vi "Append Text polymorphic.vi"   [LabVIEW 2019]
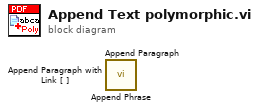
[diagram p0: block diagram]
diagram:
  n1 = call <userlib>:"Append Phrase.vi"() -> ()  [unwired: 14 in, 2 out]
  n2 = call <userlib>:"Append Paragraph.vi"() -> ()  [unwired: 14 in, 2 out]
  n3 = call <userlib>:"Append Paragraph with Link [ ].vi"() -> ()  [unwired: 14 in, 2 out]
